vi "Create Log File.vi"(8 "error in (no error)":errorcluster, 11 "appended path":path) -> (0 "error out":errorcluster)   [LabVIEW 2018, in "Mock Temperature Controller Control Panel.lvlib" / "Logging.lvlib"]
uses:
  Logging.lvlib
panel:
  out "Log file refnum out":refnum<file>
  in  "Log File Type":string="CSV"
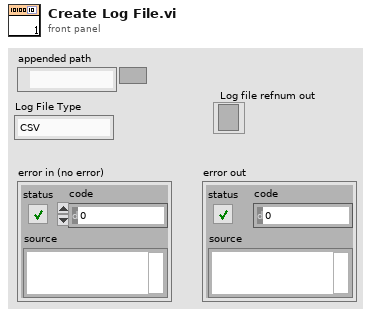
[diagram p1: front panel]
types:
  T1 = enum16{"open", "replace", "create", "open or create", "replace or create", "replace or create with confirmation"}
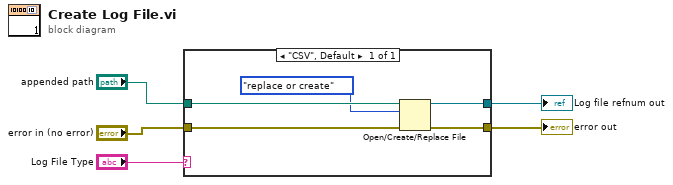
[diagram p0: block diagram]
diagram:
  n1 = case shown="\"CSV\", Default" "Log File Type" {
    tunnel: "error in (no error)" -> [w9]
    tunnel: [w7] -> w4
    tunnel: "appended path" -> [w10]
    tunnel: [w6] -> w1
    frame "CSV", Default {
      n2 = Open/Create/Replace File(file path (use dialog)=w10, error in=w9, operation (0:open)=T1."replace or create") -> (refnum out=w6:refnum<file>, error out=w7:errorcluster)  [unwired: 3 in, 1 out]
    }
  }
  "error out" <- w4
  "Log file refnum out" <- w1
